vi "toInternalIndex.vi"(1 "Square":T1={"File"=enum."d", "Rank"=enum."4"}) -> (0 "Internal index":u8)   [LabVIEW 2015, in "Chesslib.lvlib" / "Board.lvclass"]
uses:
  Board.lvclass
  typedef/Square.ctl
  typedef/File.ctl
  typedef/Rank.ctl
  Chesslib.lvlib
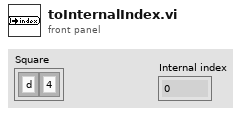
[diagram p1: front panel]
types:
  T1 = typedef "Chesslib.lvlib/Square.ctl" = cluster{"File":T2, "Rank":T3}
  T2 = typedef "Chesslib.lvlib/File.ctl" = enum8{"a", "b", "c", "d", "e", "f", "g", "h"}
  T3 = typedef "Chesslib.lvlib/Rank.ctl" = enum8{"1", "2", "3", "4", "5", "6", "7", "8"}
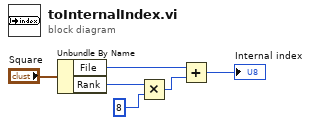
[diagram p0: block diagram]
diagram:
  n1 = Unbundle By Name("Square") -> ("File"=w2:T2, "Rank"=w5:T3)
  n2 = Multiply(x=w5, y=u8 8) -> (x*y=w3:u8)
  n3 = Add(x=w2, y=w3) -> (x+y=→"Internal index":u8)
